vi "Main.vi"() -> ()   [LabVIEW 2014]
uses:
  Global 1.vi
panel:
  out "Waveform Chart":dbl(graph)
  in  "Save":bool
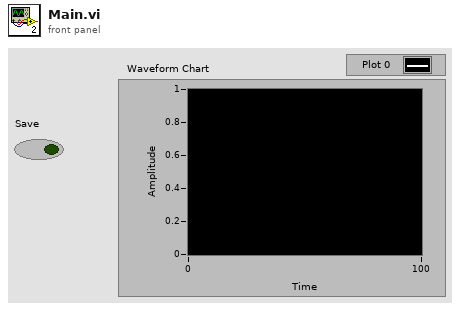
[diagram p1: front panel]
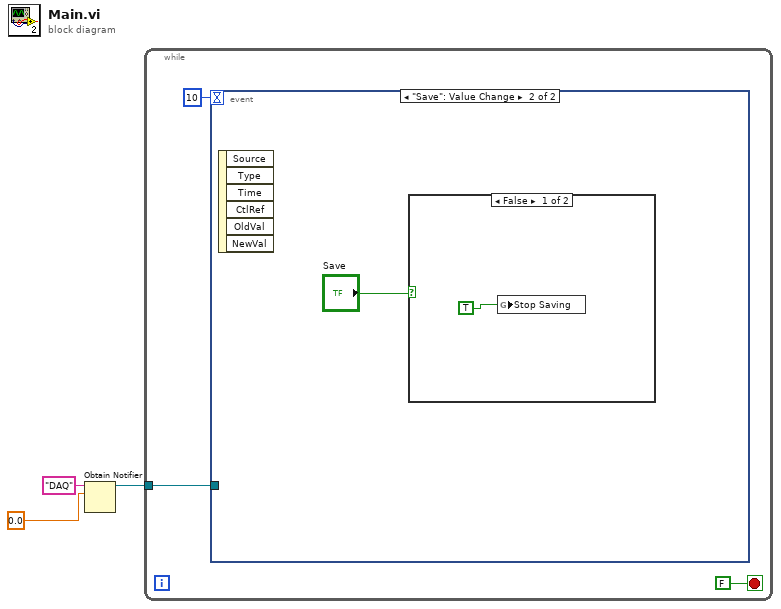
[diagram p0: block diagram]
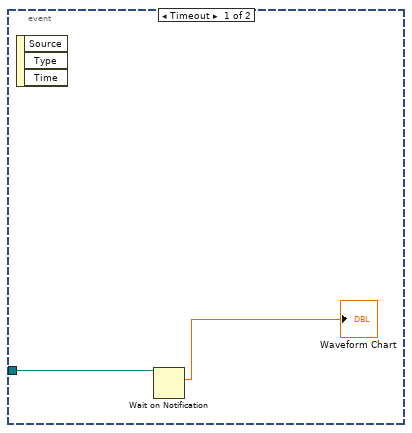
[diagram p2: hidden frame]
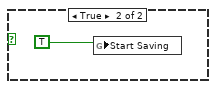
[diagram p3: hidden frame]
diagram:
  n1 = Obtain Notifier(name (unnamed)="DAQ", notification data type=0.0) -> (notifier out=w1:refnum<notifier>)  [unwired: 2 in, 2 out]
  n2 = while {
    tunnel: w1 -> [w6]
    stop <- FALSE stop-if-true
    n3 = event shown="[1] \"Save\": Value Change" {
      selector: _ -> [_ _]
      dyn-events: _ -> [_ _]
      timeout: 10 -> [_ _]
      tunnel: w6 -> [w8 _]
      event Timeout {
        n4 = event-data() -> ()  [unwired: 1 in, 3 out]
        n5 = Wait on Notification(notifier=w8) -> (notification=→"Waveform Chart":dbl)  [unwired: 3 in, 3 out]
      }
      event "Save": Value Change {
        n6 = event-data() -> ()  [unwired: 1 in, 6 out]
        n7 = case shown="False" "Save" {
          frame False {
            n8 = global write "Global 1.vi" "Stop Saving"(TRUE) -> ()
          }
          frame True {
            n9 = global write "Global 1.vi" "Start Saving"(TRUE) -> ()
          }
        }
      }
    }
  }
